vi "Eulogy User.vi"(11 "Label Text":string) -> (3 "User":string)   [LabVIEW 2017, in "Bookmark Manager.lvlib"]
uses:
  Bookmark Manager.lvlib
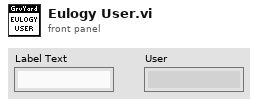
[diagram p1: front panel]
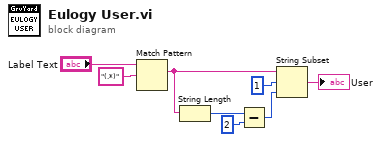
[diagram p0: block diagram]
diagram:
  n1 = Match Pattern(string="Label Text", regular expression="(.*)") -> (match substring=w7:string)  [unwired: 1 in, 3 out]
  n2 = String Length(string=w7) -> (length=w4:i32)
  n3 = Subtract(x=w4, y=2) -> (x-y=w6:i32)
  n4 = String Subset(string=w7, offset (0)=1, length (rest)=w6) -> (substring=→"User":string)
